vi "LoadConfig.vi"() -> ()   [LabVIEW 2014]
panel:
  in  "Control":T1
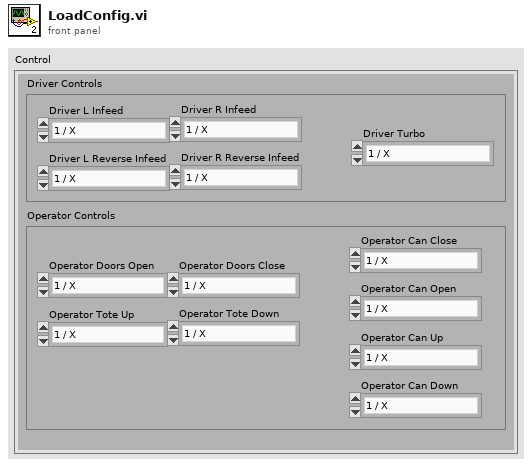
[diagram p1: front panel]
types:
  T1 = cluster{"Driver Controls":cluster{"Driver R Infeed":enum16{"1 / X", "2 / A", "3 / B", "4 / Y", "5 / Left Bumper", "6 / Right Bumper", "7 / Left Trigger", "8 / Right Trigger", "9", "10", "11 / Left Stick", "12 / Right Stick"}, "Driver L Infeed":enum16{"1 / X", "2 / A", "3 / B", "4 / Y", "5 / Left Bumper", "6 / Right Bumper", "7 / Left Trigger", "8 / Right Trigger", "9", "10", "11 / Left Stick", "12 / Right Stick"}, "Driver R Reverse Infeed":enum16{"1 / X", "2 / A", "3 / B", "4 / Y", "5 / Left Bumper", "6 / Right Bumper", "7 / Left Trigger", "8 / Right Trigger", "9", "10", "11 / Left Stick", "12 / Right Stick"}, "Driver L Reverse Infeed":enum16{"1 / X", "2 / A", "3 / B", "4 / Y", "5 / Left Bumper", "6 / Right Bumper", "7 / Left Trigger", "8 / Right Trigger", "9", "10", "11 / Left Stick", "12 / Right Stick"}, "Driver Turbo":enum16{"1 / X", "2 / A", "3 / B", "4 / Y", "5 / Left Bumper", "6 / Right Bumper", "7 / Left Trigger", "8 / Right Trigger", "9", "10", "11 / Left Stick", "12 / Right Stick"}}, "Operator Controls":cluster{"Operator Doors Open":enum16{"1 / X", "2 / A", "3 / B", "4 / Y", "5 / Left Bumper", "6 / Right Bumper", "7 / Left Trigger", "8 / Right Trigger", "9", "10", "11 / Left Stick", "12 / Right Stick"}, "Operator Doors Close":enum16{"1 / X", "2 / A", "3 / B", "4 / Y", "5 / Left Bumper", "6 / Right Bumper", "7 / Left Trigger", "8 / Right Trigger", "9", "10", "11 / Left Stick", "12 / Right Stick"}, "Operator Tote Up":enum16{"1 / X", "2 / A", "3 / B", "4 / Y", "5 / Left Bumper", "6 / Right Bumper", "7 / Left Trigger", "8 / Right Trigger", "9", "10", "11 / Left Stick", "12 / Right Stick"}, "Operator Tote Down":enum16{"1 / X", "2 / A", "3 / B", "4 / Y", "5 / Left Bumper", "6 / Right Bumper", "7 / Left Trigger", "8 / Right Trigger", "9", "10", "11 / Left Stick", "12 / Right Stick"}, "Operator Can Close":enum16{"1 / X", "2 / A", "3 / B", "4 / Y", "5 / Left Bumper", "6 / Right Bumper", "7 / Left Trigger", "8 / Right Trigger", "9", "10", "11 / Left Stick", "12 / Right Stick"}, "Operator Can Open":enum16{"1 / X", "2 / A", "3 / B", "4 / Y", "5 / Left Bumper", "6 / Right Bumper", "7 / Left Trigger", "8 / Right Trigger", "9", "10", "11 / Left Stick", "12 / Right Stick"}, "Operator Can Up":enum16{"1 / X", "2 / A", "3 / B", "4 / Y", "5 / Left Bumper", "6 / Right Bumper", "7 / Left Trigger", "8 / Right Trigger", "9", "10", "11 / Left Stick", "12 / Right Stick"}, "Operator Can Down":enum16{"1 / X", "2 / A", "3 / B", "4 / Y", "5 / Left Bumper", "6 / Right Bumper", "7 / Left Trigger", "8 / Right Trigger", "9", "10", "11 / Left Stick", "12 / Right Stick"}}}
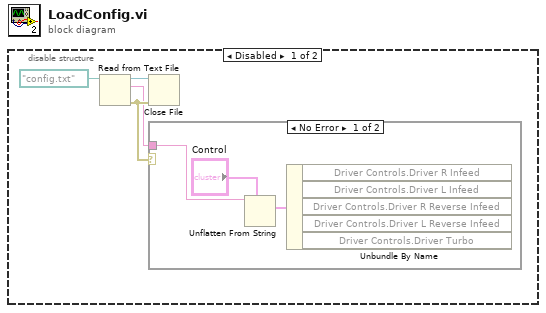
[diagram p0: block diagram]
diagram:
  n1 = disable-structure shown="Disabled" {
    frame Disabled {
      n2 = Read from Text File(file (use dialog)=path "/config.txt" ("file path (use dialog)")) -> (refnum out=w3:refnum<file>, text=w1:string, error out=w2:errorcluster)  [unwired: 3 in, 1 out]
      n3 = Close File(refnum=w3, error in=w2) -> ()  [unwired: 2 out]
      n4 = case shown="No Error" w2 {
        tunnel: w1 -> [w7 _]
        frame No Error {
          n5 = Unflatten From String(type="Control", binary string=w7) -> (value=w5:T1)  [unwired: 3 in, 2 out]
          n6 = Unbundle By Name(w5) -> ()  [unwired: 5 out]
        }
        frame Error {
        }
      }
    }
    frame Enabled {
    }
  }
